vi "SIAM-send.vi"(5 "Values":i32[](array[numeric]), 7 "connection ID":refnum<k5>, 8 "error in (no error)":errorcluster, 10 "Script":T2(array[cluster])=[{"Delay 10µs"=0, "command"=4027514895, "P0"=5, "P1"=0, "P2"=0, "P3"=0, "P4"=0, "P5-ticket"=0, "comment"=""}] {"command" format="%x" items=["end_no_ticket"=4027514895, "end_ticket"=4027518991, "NoOp"=4026531840, "Read ticks"=4026535936, "Read ticks to var"=4026535938, "Read IP"=4043313152, "Read IP into var"=4043313154, "Set IP from var"=4043309059, "Set IP from var, relative"=4043313155, "branchRel_if_equal"=4043374849, "decrement_branchRel_if_equal"=4043374945, "decrement_branchRel_if_greaterequal"=4043375201, "decrement_branchRel_if_greaterequal_withTicket"=4043379297, "decrement_branchRel_if_smaller"=4043375457, "increment_branchRel_if_smaller"=4043375473, "readVar"=4060090368, "writeVar"=4060086273, "copyVar0_from_var1"=4060086275, "math_addToVariable"=4076863488, "math_addVToVariable"=4076863489, "math_subToVariable"=4076863490, "math_subVToVariable"=4076863491, "math_multToVariable"=4076863492, "math_multvToVariable"=4076863493, "math_divideToVariable"=4076863494, "math_divideVToVariable"=4076863495, "math_modToVariable"=4076863496, "math_modVToVariable"=4076863497, "logic_and"=4093640704, "logic_or"=4093640706, "logic_xor"=4093640708, "bitshift"=4093640712, "I2C-write"=335544337, "I2C-read"=335548433, "Cam-SPI-write"=3254779905, "UART0-VC-Baud-write"=469958673, "UART0-VC-Baud-read"=469962768, "UART0-VC-write"=469762065, "UART0-VC-write-Var"=469762067, "UART0-VC-read-availabe-bytes-to-var"=470355970, "UART0-VC-read-availabe-bytes"=470355984, "UART0-VC-read-skip-bytes"=469831681, "UART0-VC-read"=469766160, "UART0-VC-read-Var"=469766162, "UART1-TSM-Baud-write"=486735889, "UART1-TSM-Baud-read"=486739984, "UART1-TSM-write"=486539281, "UART1-TSM-write-Var"=486539283, "UART1-TSM-read-availabe-bytes-to-var"=487133186, "UART1-TSM-read-availabe-bytes"=487133200, "UART1-TSM-read-skip-bytes"=486604801, "UART1-TSM-read-skip-bytes"=486608897, "UART1-TSM-read"=486543376, "UART1-TSM-read-Var"=486543378, "UART2-Laser-Baud-write"=503513105, "UART2-Baud-read"=503517200, "UART2-write"=503316497, "UART2-write-Var"=503316499, "UART2-read-availabe-bytes-to-var"=503910402, "UART2-read-availabe-bytes"=503910416, "UART2-read-skip-bytes"=503386113, "UART2-read"=503320592, "UART2-read-Var"=503320594, "UART3-Baud-write"=520290321, "UART3-Baud-read"=520294416, "UART3-write"=520093713, "UART3-write-Var"=520093715, "UART3-read-availabe-bytes-to-var"=520687618, "UART3-read-availabe-bytes"=520687632, "UART3-read-skip-bytes"=520163329, "UART3-read"=520097808, "UART3-read-Var"=520097810, "IO-read_bank0"=3489665024, "IO-write_bank0"=3489660929, "IO-read_bank1"=3506442240, "IO-write_bank1"=3506438145, "DA0-0_LED365"=2684354561, "DA0-1_LED385"=2685403137, "DA0-2_LED440"=2686451713, "DA0-3_LED470"=2687500289, "DA0-4_LED510"=2688548865, "DA0-5_LED550"=2689597441, "DA0-6_LED590"=2690646017, "DA0-7_LED640"=2691694593, "DA1-0_LED-R"=2701131777, "DA1-1_LED-G"=2702180353, "DA1-2_LED-B"=2703228929, "DA1-3_LED-AF"=2704277505, "DA1-4"=2705326081, "DA1-5"=2706374657, "DA1-6"=2707423233, "DA1-7"=2708471809, "DA2-Laser0"=2717908993, "DA2-Laser1"=2718957569, "DA2-Laser2"=2720006145, "DA2-Laser3"=2721054721, "DA2-Laser4"=2722103297, "Analog-read_AD0-0"=2818576384, "Analog-read-store_AD0-0"=2818572290, "AF-Register-transfer r/w"=2835349505, "AF-Register-read"=2835353600, "AF-Register-read-to-var"=2835353602, "AF-Transfer-from-var"=2835349507, "IO-delay_bank0"=3489923073, "IO-delay_bank0_fromVar"=3489923075, "read_cam_clock"=3289124864, "store_cam_clock"=3289120770, "read_cam_phase"=3289190400, "store_cam_phase"=3289186306, "store_cam_phase-t"=3289190402, "r_cam1_NHS"=3254980608, "w_cam1_NHS"=3254976513, "r_cam1_NVS"=3255046144, "w_cam1_NVS"=3255042049, "r_cam1_npx"=3255111680, "w_cam1_npx"=3255107585, "r_cam1_npy"=3255177216, "w_cam1_npy"=3255173121, "r_cam1_xhswait"=3255439360, "w_cam1_xhswait"=3255435265, "r_cam1_xvs_wait"=3255504896, "w_cam1_xvs_wait"=3255500801, "r_cam1_framcounter"=3255570432, "r_cam1_line"=3255635968, "r_cam1_xhs-counter"=3255701504, "r_cam2_NHS"=3271757824, "w_cam2_NHS"=3271753729, "r_cam2_NVS"=3271823360, "w_cam2_NVS"=3271819265, "r_cam2_npx"=3271888896, "w_cam2_npx"=3271884801, "r_cam2_npy"=3271954432, "w_cam2_npy"=3271950337, "r_cam2_xvs_wait"=3272282112, "w_cam2_xvs_wait"=3272278017, "r_cam2_framcounter"=3272347648, "r_cam2_line"=3272413184, "r_cam2_xhs-counter"=3272478720, "start TMSI"=102694919, "set_1Galvo"=101712113, "set_x-Galvo"=102760689, "set_y-Galvo"=103809265, "set_z-Fokus"=104857841, "set_1Galvo_position-only"=101711937, "set_x-Galvo_position-only"=102760513, "set_y-Galvo_position-only"=103809089, "set_z-Fokus_position-only"=104857665, "set_x-Galvo_position-only_ticket"=102764609, "set_y-Galvo_position-only_ticket"=103813185, "set_z-Fokus_position-only_ticket"=104861761, "set_1Galvo_relativ-only"=101712001, "set_x-Galvo_relativ-only"=102760577, "set_y-Galvo_relativ-only"=103809153, "set_z-Fokus_relativ-only"=104857729, "set_1Galvo_speed-only"=101711905, "set_x-Galvo_speed-only"=102760481, "set_y-Galvo_speed-only"=103809057, "set_z-Fokus_speed-only"=104857633, "set_1Galvo_acc-only"=101711889, "set_x-Galvo_acc-only"=102760465, "set_y-Galvo_acc-only"=103809041, "set_z-Fokus_acc-only"=104857617, "read_1Galvo_ticket"=101716032, "read_x-Galvo_ticket"=102764608, "read_y-Galvo_ticket"=103813184, "read_z-Focus_ticket"=104861760, "x-Galvo_pos_fromVar"=102760515, "y-Galvo_pos_fromVar"=103809091, "z-Focus_pos_fromVar"=104857667, "Servo0"=67108865, "Servo0-enable"=68091911, "Servo0-disable"=68091919, "Servo1"=68157441, "Servo1-enable"=69140487, "Servo1-disable"=69140495, "Servo2-enable"=70189063, "Servo2"=69206017, "Servo3-enable"=71237639, "Servo3"=70254593, "x-ssi-init"=202309639, "x-ssi-disable"=202309647, "x-ssi-Bits"=201523201, "x-ssi-Read"=201330688, "x-ssi-ReadToVar"=201326594, "x-ssi-ReadToVar-ticket"=201330690, "y-ssi-init"=203358215, "y-ssi-disable"=203358223, "y-ssi-Bits"=202571777, "y-ssi-Read"=202379264, "y-ssi-ReadToVar"=202375170, "y-ssi-ReadToVat-ticket"=202379266]}, 11 "command":T3) -> (0 "error out":errorcluster, 2 "Status":enum16{"unknown", "idle", "running", ""}(ring))   [LabVIEW 2011]
uses:
  SIAM-send.ctl
  SIAM_command.ctl
panel:
  # "store locally to allow usage from other vi's"
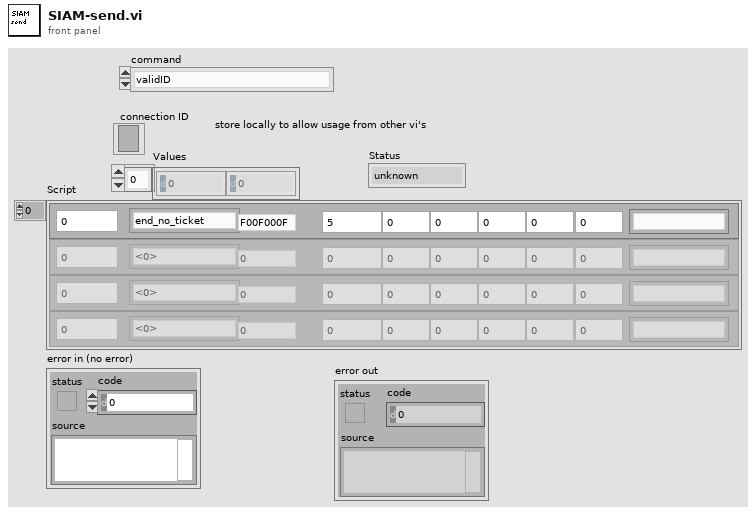
[diagram p1: front panel]
types:
  T1 = typedef "SIAM_command.ctl" = u32
  T2 = cluster{"Delay 10µs":u32, "command":T1, "P0":i32, "P1":i32, "P2":i32, "P3":i32, "P4":i32, "P5-ticket":i32, "comment":string}[]
  T3 = typedef "SIAM-send.ctl" = enum16{"validID", "storeID", "enable", "rundirect", "sendlist", "run", "stop", "readRegister", "sendValue", "storeStatus"}
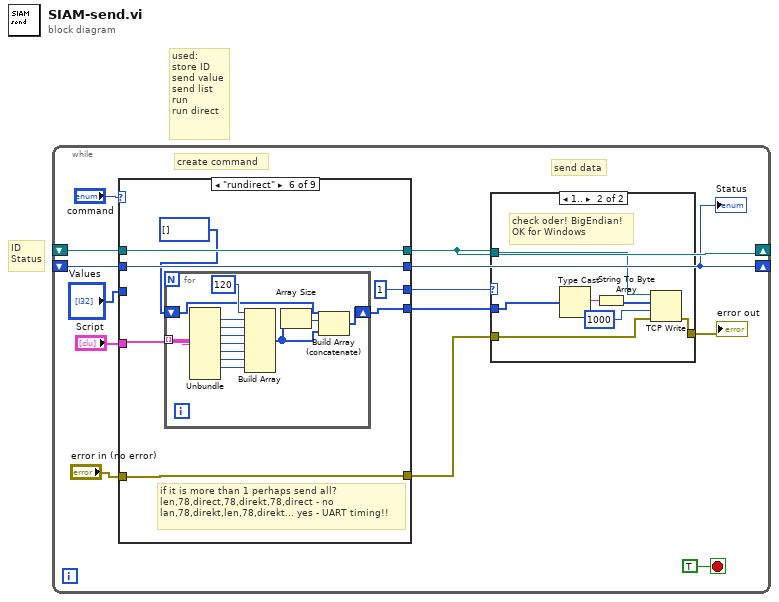
[diagram p0: block diagram]
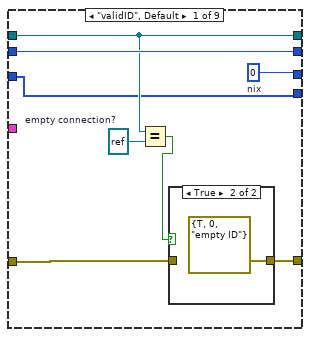
[diagram p3: hidden frame]
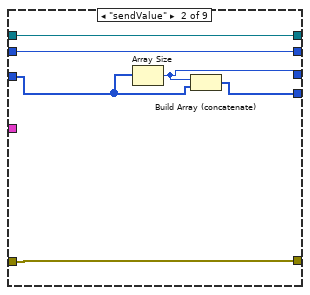
[diagram p5: hidden frame]
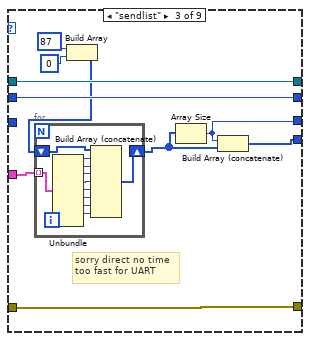
[diagram p6: hidden frame]
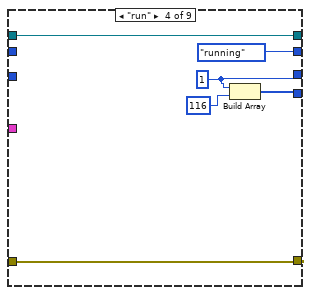
[diagram p7: hidden frame]
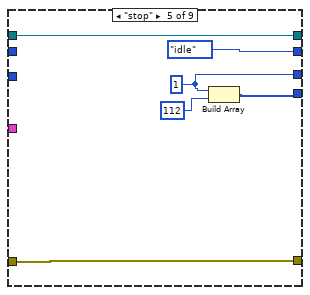
[diagram p8: hidden frame]
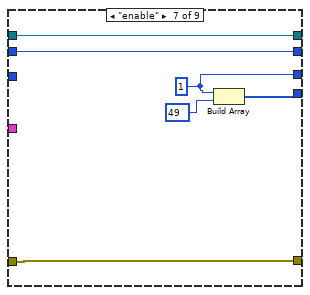
[diagram p9: hidden frame]
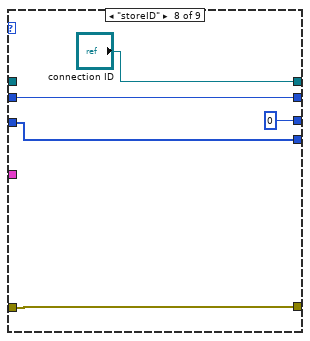
[diagram p10: hidden frame]
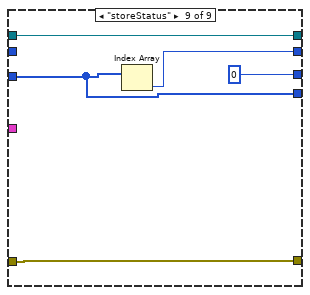
[diagram p11: hidden frame]
diagram:
  # "used: \nstore ID\nsend value\nsend list\nrun\nrun direct"
  # "ID\nStatus"
  n1 = while {
    shift-right: [w5] -> _
    shift-left: _ -> [w11]
    shift-right: [w3] -> _
    shift-left: _ -> [w10]
    stop <- TRUE stop-if-true
    # "send data"
    # "create command"
    n2 = case shown="\"rundirect\"" "command" {
      tunnel: [w28 w36 w47 w64 w69 w77 w96 "connection ID" w106] -> w5
      tunnel: w11 -> [w28 w36 w47 w64 w69 w77 w96 _ w106]
      tunnel: [w29 w37 w46 enum16{"unknown", "idle", "running", ""}."running" ("Status") enum16{"unknown", "idle", "running", ""}."idle" ("Status") w76 w95 w100 w104] -> w3
      tunnel: w10 -> [w29 w37 w46 _ _ w76 w95 w100 _]
      tunnel: "Script" -> [_ _ w44 _ _ w74 _ _ _]
      tunnel: "error in (no error)" -> [w25 w35 w45 w63 w68 w75 w94 w99 w105]
      tunnel: [w24 w35 w45 w63 w68 w75 w94 w99 w105] -> w6
      tunnel: [w22 w33 w40 w61 w66 w72 w91 w97 w102] -> w4
      tunnel: "Values" -> [w22 w34 _ _ _ _ _ w97 w102]
      tunnel: [w23 w32 w38 w59 w65 u32 1 ("nix") w92 u32 0 ("nix") u32 0 ("nix")] -> w1
      frame "validID", Default {
        w23 = u32 0  # nix
        w27 = refnum<k5> refnum  # empty connection?
        n3 = Equal?(x=w28, y=w27) -> (x = y?=w26:bool)
        n4 = case shown="True" w26 {
          tunnel: w25 -> [w30 _]
          tunnel: [w30 errorcluster {"status"=TRUE, "code"=0, "source"="empty ID"} ("error in (no error)")] -> w24
          frame False {
          }
          frame True {
          }
        }
      }
      frame "sendValue" {
        n5 = Array Size(array=w34) -> (size(s)=w32:i32)
        n6 = Build Array (concatenate)(w32, w34) -> (w33:i32[])
      }
      frame "sendlist" {
        # "sorry direct no time\ntoo fast for UART"
        n7 = Build Array(87, u32 0 ("element")) -> (w39:u32[])
        n8 = for {
          tunnel: w44 -> [w58] mode=indexing
          shift-right: [w48] -> w41
          shift-left: w39 -> [w49]
          n9 = Unbundle(w58) -> ("Delay 10µs"=w57:u32, "command"=w56:T1, "P0"=w55:i32, "P1"=w54:i32, "P2"=w53:i32, "P3"=w52:i32, "P4"=w51:i32, "P5-ticket"=w50:i32)  [unwired: 1 out]
          n10 = Build Array (concatenate)(w49, w57, w56, w55, w54, w53, w52, w51, w50) -> (w48:T1[])
        }
        n11 = Array Size(array=w41) -> (size(s)=w38:i32)
        n12 = Build Array (concatenate)(w38, w41) -> (w40:T1[])
      }
      frame "run" {
        w59 = u32 1 ("nix")
        n13 = Build Array(w59, 116) -> (w61:u32[])
      }
      frame "stop" {
        w65 = u32 1 ("nix")
        n14 = Build Array(w65, 112) -> (w66:u32[])
      }
      frame "rundirect" {
        # "if it is more than 1 perhaps send all?\nlen,78,direct,78,direkt,78,direct - no\nlan,78,direkt,len,78,direkt... yes - UART timing!!"
        n15 = for {
          tunnel: w74 -> [w90] mode=indexing
          shift-right: [w79] -> w72
          shift-left: u32[] [] -> [w78]
          n16 = Unbundle(w90) -> ("command"=w89:T1, "P0"=w88:i32, "P1"=w87:i32, "P2"=w86:i32, "P3"=w85:i32, "P4"=w84:i32, "P5-ticket"=w83:i32)  [unwired: 2 out]
          n17 = Build Array(120, w89, w88, w87, w86, w85, w84, w83) -> (w80:T1[])
          n18 = Array Size(array=w80) -> (size(s)=w81:i32)
          n19 = Build Array (concatenate)(w78, w81, w80) -> (w79:T1[])
        }
      }
      frame "enable" {
        w92 = u32 1 ("nix")
        n20 = Build Array(w92, 49) -> (w91:u32[])
      }
      frame "storeID" {
      }
      frame "storeStatus" {
        n21 = Index Array(array=w102) -> (element=w104:i32)  [unwired: 1 in]
      }
    }
    "Status" <- w3
    n22 = case shown="1.." w1 {
      tunnel: [w14 w21] -> w7
      tunnel: w6 -> [w14 w20]
      tunnel: w5 -> [_ w19]
      tunnel: w4 -> [_ w15]
      frame 0, Default {
        # "nothing to send"
      }
      frame 1.. {
        # "check oder! BigEndian!\nOK for Windows"
        n23 = Type Cast(x=w15) -> (*(type *) &x=w17:string)  [unwired: 1 out]
        n24 = String To Byte Array(string=w17) -> (unsigned byte array=w16:u8[])
        n25 = TCP Write(connection ID=w19, data in=w16, error in (no error)=w20, 9:1000 ("timeout ms (25000)")) -> (error out=w21:errorcluster)  [unwired: 2 out]
      }
    }
    "error out" <- w7
  }
